vi "zmq_FBINJ_sim.vi"() -> ()   [LabVIEW 2014]
uses:
  <vilib>/addons/zeromq/socket_type.ctl
  <vilib>/addons/zeromq/zmq_context.lvclass
  <vilib>/addons/zeromq/zmq_socket.lvclass
  <vilib>/addons/zeromq/zeromq.lvlib
panel:
  in  "Source":u16(ring) items=["Laptop", "Campus"]
  out "Status":string="Complete"
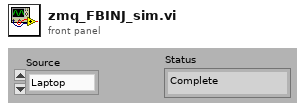
[diagram p1: front panel]
types:
  T1 = typedef "zeromq.lvlib/socket_type.ctl" = enum8{"ZMQ_PAIR", "ZMQ_PUB", "ZMQ_SUB", "ZMQ_REQ", "ZMQ_REP", "ZMQ_DEALER", "ZMQ_ROUTER", "ZMQ_PULL", "ZMQ_PUSH", "ZMQ_XPUB", "ZMQ_XSUB"}
  T2 = enum16{"big-endian, network order", "native, host order", "little-endian"}
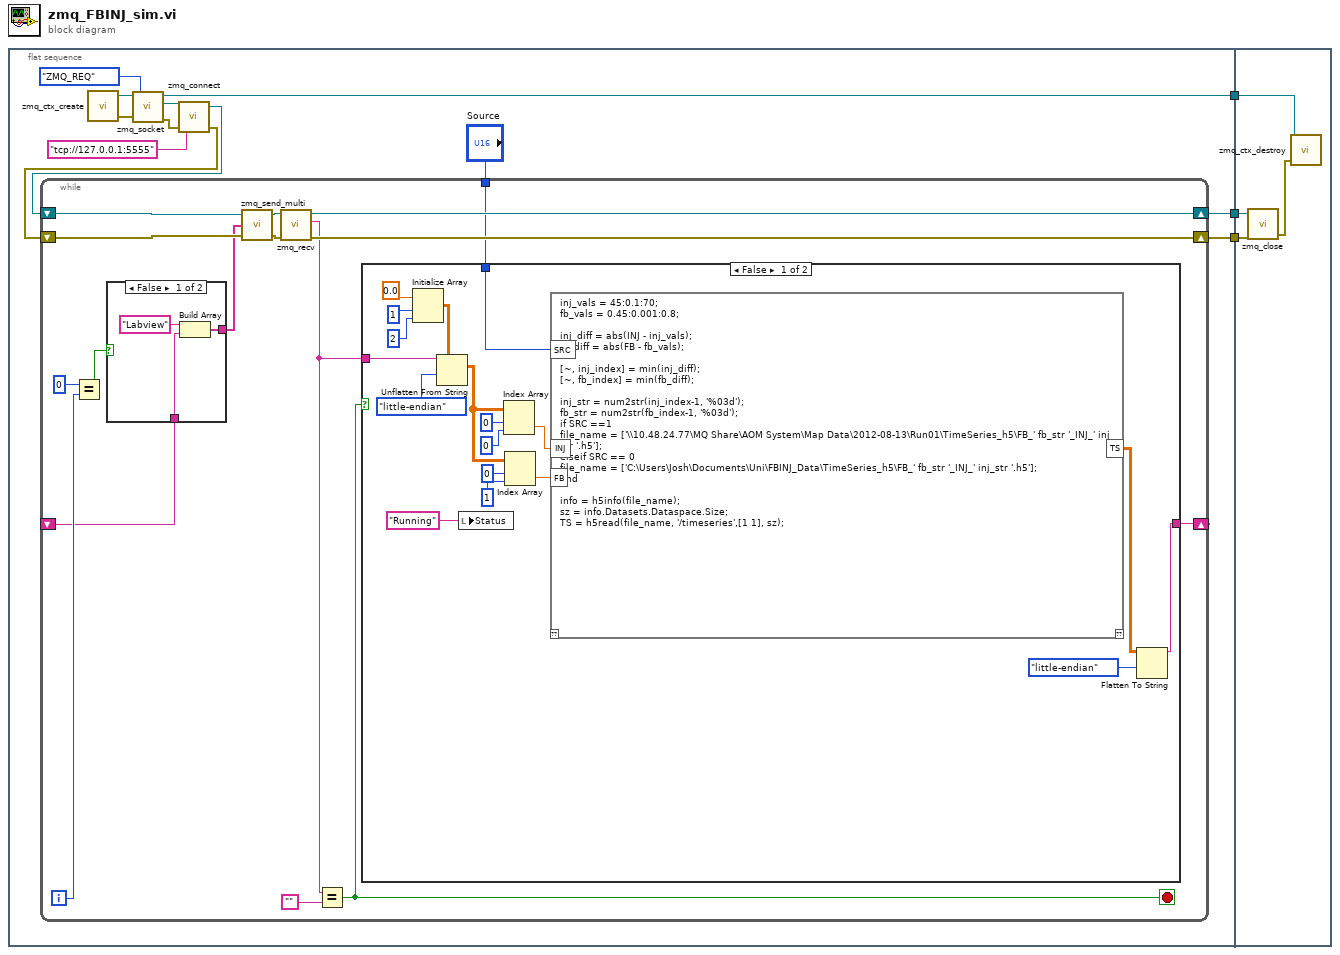
[diagram p0: block diagram]
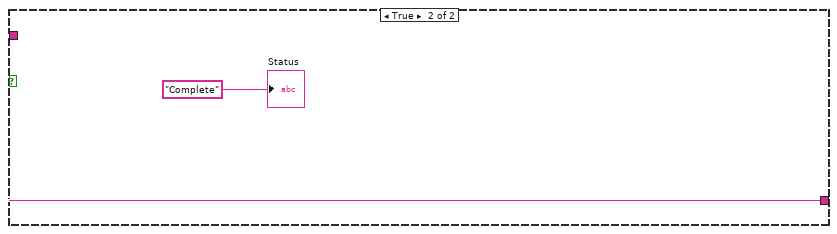
[diagram p2: hidden frame]
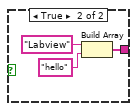
[diagram p3: hidden frame]
diagram:
  n1 = flat-sequence {
    tunnel: [w11] -> w3
    tunnel: [w5] -> w2
    tunnel: [w6] -> w1
    tunnel: w3 -> [w61]
    tunnel: w2 -> [w59]
    tunnel: w1 -> [w58]
    frame #0 {
      n2 = call <vilib>:"zmq_ctx_create.vi"() -> ("error out"=w10:errorcluster, "context out"=w15:refnum<class "zmq_context.lvclass">)  [unwired: 4 in]
      n3 = call <vilib>:"zmq_socket.vi"("error in"=w10, "socket type"=socket_type."ZMQ_REQ", "context in"=w15) -> ("error out"=w14:errorcluster, "socket out"=w13:refnum<class "zmq_socket.lvclass">, "context out"=w11:refnum<class "zmq_context.lvclass">)  [unwired: 2 in]
      n4 = call <vilib>:"zmq_connect.vi"("error in"=w14, "endpoint"="tcp://127.0.0.1:5555", "socket in"=w13) -> ("error out"=w7:errorcluster, "socket out"=w12:refnum<class "zmq_socket.lvclass">)  [unwired: 1 in]
      n5 = while {
        shift-right: [w26] -> w5
        shift-left: w12 -> [w31]
        shift-right: [w27] -> w6
        shift-left: w7 -> [w30]
        shift-right: [w25] -> _
        shift-left: _ -> [w21]
        tunnel: "Source" -> [w16]
        i -> [w24]
        stop <- w18 stop-if-true
        n6 = Equal?(x=0, y=w24) -> (x = y?=w22:bool)
        n7 = case shown="False" w22 {
          tunnel: [w53 w57] -> w17
          tunnel: w21 -> [w52 _]
          frame False {
            n8 = Build Array("Labview", w52) -> (w53:string[])
          }
          frame True {
            n9 = Build Array("Labview", "hello" ("element")) -> (w57:string[])
          }
        }
        n10 = call <vilib>:"zmq_send_multi.vi"("error in"=w30, "parts"=w17, "socket in"=w31) -> ("error out"=w28:errorcluster, "socket out"=w29:refnum<class "zmq_socket.lvclass">)  [unwired: 1 in]
        n11 = call <vilib>:"zmq_recv.vi"("error in"=w28, "socket in"=w29) -> ("error out"=w27:errorcluster, "data"=w19:string, "socket out"=w26:refnum<class "zmq_socket.lvclass">)  [unwired: 3 in, 2 out]
        n12 = Equal?(x=w19, y="") -> (x = y?=w18:bool)
        n13 = case shown="False" w18 {
          tunnel: [w36 w51] -> w25
          tunnel: w19 -> [w35 w51]
          tunnel: w16 -> [w32 _]
          frame False {
            n14 = Initialize Array(0.0, 1 ("dimension size"), 2 ("dimension size")) -> (w45:dbl[][])
            n15 = Unflatten From String(type=w45, binary string=w35, byte order (0:big-endian, network order)=T2."little-endian") -> (value=w42:dbl[][])  [unwired: 2 in, 2 out]
            n16 = local write "Status"("Running" ("Status")) -> ()
            n17 = Index Array(array=w42, index (row)=0 ("disabled index (row)"), index (col)=0 ("disabled index (col)")) -> (element=w41:dbl)
            n18 = Index Array(array=w42, index (row)=0 ("disabled index (row)"), index (col)=1 ("disabled index (col)")) -> (element=w38:dbl)
            n19 = script code="inj_vals = 45:0.1:70;\nfb_vals = 0.45:0.001:0.8;\n\ninj_diff = abs(INJ - inj_vals);\nfb_diff = abs(FB - fb_vals);\n\n[~, inj_index] = min(inj_diff);\n[~, fb_index] = min(fb_diff);\n\ninj_str = num2str(inj_index-1, '%03d');\nfb_str = num2str(fb_index-1, '%03d');\nif SRC ==1\nfile_name = ['\\\\10.48.24.77\\MQ Share\\AOM System\\Map Data\\2012-08-13\\Run01\\TimeSeries_h5\\FB_' fb_str '_INJ_' inj_str '.h5'];\nelseif SRC == 0\nfile_name = ['C:\\Users\\Josh\\Documents\\Uni\\FBINJ_Data\\TimeSeries_h5\\FB_' fb_str '_INJ_' inj_str '.h5'];\nend\n\ninfo = h5info(file_name);\nsz = info.Datasets.Dataspace.Size;\nTS = h5read(file_name, '/timeseries',[1 1], sz);"("INJ"=w41, "FB"=w38, "SRC"=w32) -> ("TS"=w33:dbl[][])  [unwired: 1 in, 1 out]
            n20 = Flatten To String(anything=w33, byte order (0:big-endian, network order)=T2."little-endian") -> (data string=w36:string)  [unwired: 2 in, 2 out]
          }
          frame True {
            "Status" <- "Complete"
          }
        }
      }
    }
    frame #1 {
      n21 = call <vilib>:"zmq_close.vi"("error in"=w58, "socket"=w59) -> ("error out"=w60:errorcluster)  [unwired: 3 in]
      n22 = call <vilib>:"zmq_ctx_destroy.vi"("error in"=w60, "context in"=w61) -> ()  [unwired: 3 in, 1 out]
    }
  }
